vi "ke37xx Get TSP Script Catalog.vi"(8 "error in (no error)":errorcluster, 11 "VISA Resource Name":refnum<visa-resource-name>) -> (0 "error out":errorcluster, 2 "Stored TSP Script Names":string[](array[string]), 3 "VISA Resource Name Out":refnum<visa-resource-name>)   [LabVIEW 2009, in "Keithley 3700 Series.lvlib"]
doc: "This VI returns the names of the user scripts stored on the instrument."
uses:
  <instrlib>/Keithley 3706/Keithley 3700 Series.lvlib
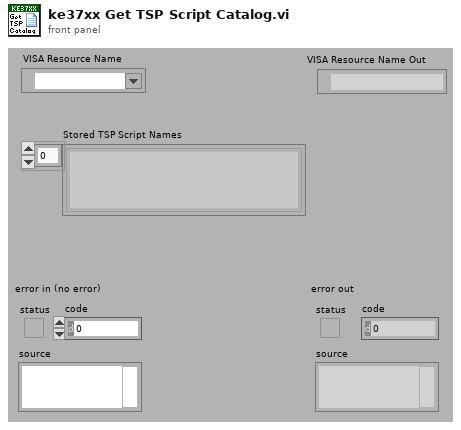
[diagram p1: front panel]
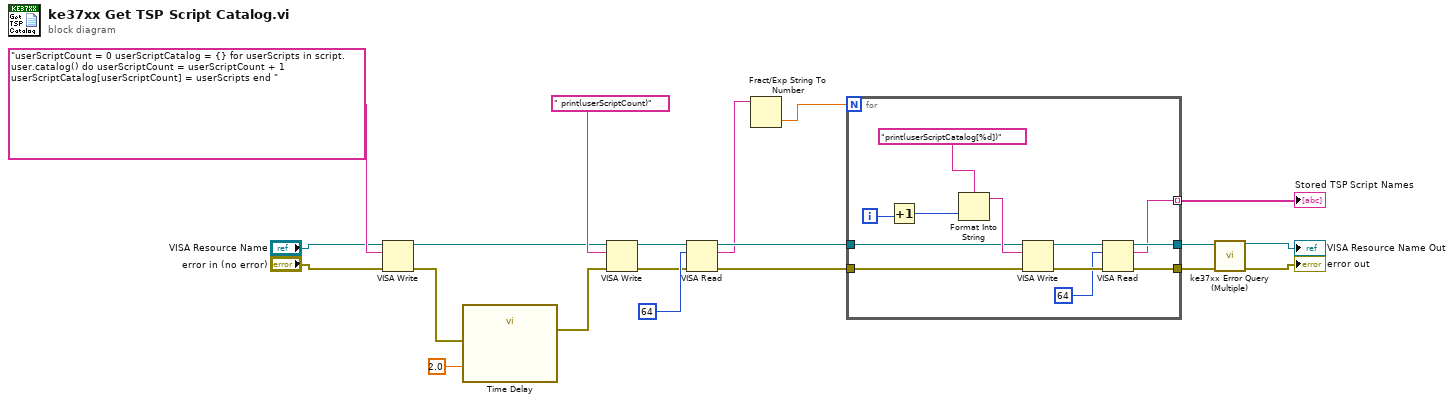
[diagram p0: block diagram]
diagram:
  n1 = VISA Write(VISA resource name="VISA Resource Name", write buffer="userScriptCount = 0 userScriptCatalog = {} for userScripts in script.user.catalog() do userScriptCount = userScriptCount + 1 userScriptCatalog[userScriptCount] = userScripts end ", error in (no error)="error in (no error)") -> (VISA resource name out=w6:refnum<visa-resource-name>, error out=w5:errorcluster)  [unwired: 1 out]
  n2 = call "Time Delay"("error in (no error)"=w5, "Delay Time (s)"=2.0) -> ("error out"=w4:errorcluster)  [unwired: 9 in]
  n3 = VISA Write(VISA resource name=w6, write buffer=" print(userScriptCount)", error in (no error)=w4) -> (VISA resource name out=w9:refnum<visa-resource-name>, error out=w8:errorcluster)  [unwired: 1 out]
  n4 = VISA Read(VISA resource name=w9, byte count=64, error in (no error)=w8) -> (VISA resource name out=w15:refnum<visa-resource-name>, read buffer=w2:string, error out=w16:errorcluster)  [unwired: 1 out]
  n5 = Fract/Exp String To Number(string=w2) -> (number=w1:dbl)  [unwired: 3 in, 1 out]
  n6 = for {
    N: w1 -> [_]
    tunnel: w16 -> [w28]
    tunnel: w15 -> [w27]
    tunnel: [w23] -> w14
    tunnel: [w22] -> w13
    tunnel: [w21] -> w12 mode=indexing
    i -> [w32]
    n7 = Increment(x=w32) -> (x+1=w31:i32)
    n8 = Format Into String(format string="print(userScriptCatalog[%d])", w31) -> (resulting string=w29:string)  [unwired: 2 in, 1 out]
    n9 = VISA Write(VISA resource name=w27, write buffer=w29, error in (no error)=w28) -> (VISA resource name out=w26:refnum<visa-resource-name>, error out=w25:errorcluster)  [unwired: 1 out]
    n10 = VISA Read(VISA resource name=w26, byte count=64, error in (no error)=w25) -> (VISA resource name out=w23:refnum<visa-resource-name>, read buffer=w21:string, error out=w22:errorcluster)  [unwired: 1 out]
  }
  "Stored TSP Script Names" <- w12
  n11 = call <instrlib>:"ke37xx Error Query (Multiple).vi"("VISA resource name"=w14, "error in (no error)"=w13) -> ("VISA resource name out"=→"VISA Resource Name Out":refnum<visa-resource-name>, "error out"=→"error out":errorcluster)  [unwired: 12 out]
